vi "Configure Counter New Setpoint.vi"(8 "error in (no error)":errorcluster, 9 "Counter Setpoint (0%)":dbl min=0.0 max=100.0 step=1.0 format="%#g", 10 "Node (3)":u8=3 caption="Node" min=3 max=128 step=1, 11 "VISA resource name":refnum<visa-resource-name>) -> (0 "error out":errorcluster, 3 "VISA resource name out":refnum<visa-resource-name>)   [LabVIEW 2024, in "Bronkhorst FLOW-BUS.lvlib"]
doc: "Configures the new/safe setpoint value that will be set when a counter limit/batch situation (until reset) occurs. To enable this use the <b>Configure Counter Setpoint Mode</b> VI."
uses:
  Bronkhorst FLOW-BUS.lvlib
  Private/FLOW-BUS RW.ctl
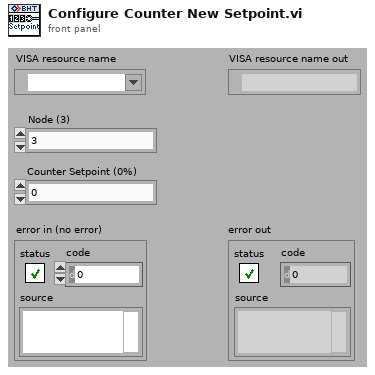
[diagram p1: front panel]
types:
  T1 = typedef "Bronkhorst FLOW-BUS.lvlib/FLOW-BUS RW.ctl" = cluster{"Node Address (3)":u8, "Communication Command":enum16{"Status message", "Send parameter with destination address and 00 response", "Send parameter with destination address", "Request parameter"}, "Process (0)":u16, "Parameter (0)":u16, "Data Type (0: Character)":enum16{"Character", "Integer", "Float or Long", "String"}, "Data for Char, Int, or Long (0)":u32, "Data for Float (0)":sgl, "Data for String":string, "Length of Requested String (0)":u8}
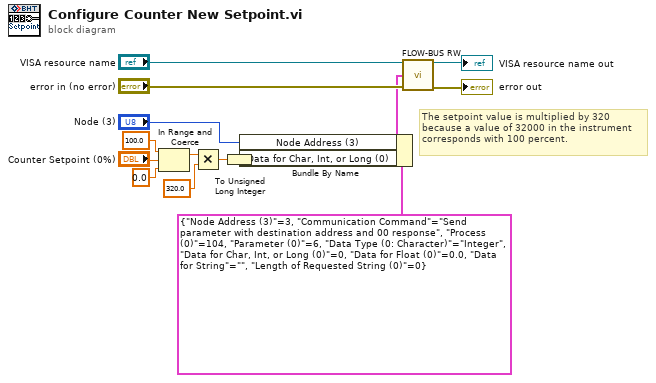
[diagram p0: block diagram]
diagram:
  # "The setpoint value is multiplied by 320\nbecause a value of 32000 in the instrument\ncorresponds with 100 percent."
  n1 = In Range and Coerce(upper limit=100.0, x="Counter Setpoint (0%)", lower limit=0.0) -> (coerced(x)=w10:dbl)  [unwired: 1 out]
  n2 = Multiply(x=w10, y=320.0) -> (x*y=w8:dbl)
  n3 = To Unsigned Long Integer(number=w8) -> (unsigned 32bit integer=w9:u32)
  n4 = Bundle By Name(cluster=T1 {"Node Address (3)"=3, "Communication Command"=enum."Send parameter with destination address and 00 response", "Process (0)"=104, "Parameter (0)"=6, "Data Type (0: Character)"=enum."Integer", "Data for Char, Int, or Long (0)"=0, "Data for Float (0)"=0.0, "Data for String"="", "Length of Requested String (0)"=0} ("FLOW-BUS Command Settings"), "Node Address (3)"="Node (3)", "Data for Char, Int, or Long (0)"=w9) -> (w2:T1)
  n5 = call "FLOW-BUS RW.vi"("VISA resource name"="VISA resource name", "FLOW-BUS Command Settings"=w2, "error in (no error)"="error in (no error)") -> ("VISA resource name out"=→"VISA resource name out":refnum<visa-resource-name>, "error out"=→"error out":errorcluster)  [unwired: 8 in, 3 out]
